vi "Port Open (SubVI).vi"(0 "VISA Refnum in":refnum<visa-resource-name>) -> (1 "VISA Refnum out":refnum<visa-resource-name>, 2 "error out":errorcluster)   [LabVIEW 2017]
doc: "by Tanguy BOULARD"
uses:
  <vilib>/Instr/_visa.llb/VISA Configure Serial Port (Instr).vi
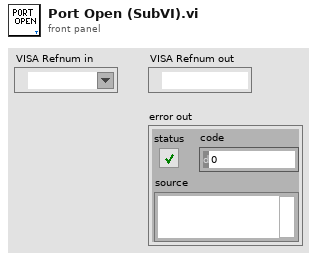
[diagram p1: front panel]
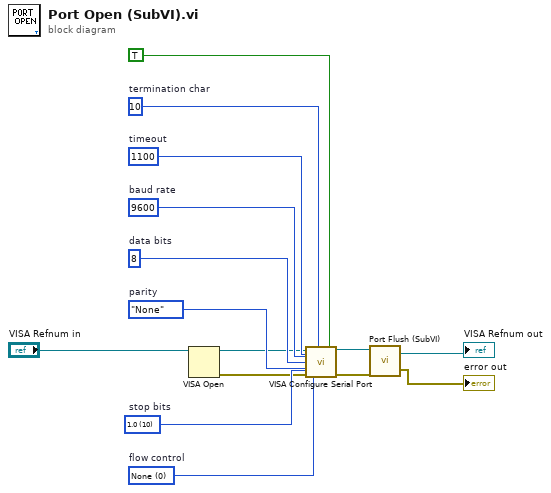
[diagram p0: block diagram]
diagram:
  w14 = u16 0 items=["None", "XON/XOFF", "RTS/CTS", "XON/XOFF & RTS/CTS", "DTR/DSR", "XON/XOFF & DTR/DSR"]  # flow control
  w13 = u16 10 items=["1.0"=10, "1.5"=15, "2.0"=20]  # stop bits
  w12 = u16 8  # data bits
  w11 = enum16{"None", "Odd", "Even", "Mark", "Space"}."None"  # parity
  w10 = u32 9600  # baud rate
  w8 = u32 1100  # timeout
  w9 = u8 10  # termination char
  n1 = VISA Open(VISA resource name="VISA Refnum in") -> (VISA resource name=w1:refnum<visa-resource-name>, error out=w2:errorcluster)  [unwired: 4 in]
  n2 = call-poly "VISA Configure Serial Port"("VISA resource name"=w1, "timeout (10sec)"=w8, "termination char\n(0xA = '\\n' = LF)"=w9, "Enable Termination\nChar (T)"=TRUE ("Enable Termination\nChar (T)"), "baud rate (9600)"=w10, "data bits (8)"=w12, "parity (0:none)"=w11, "error in (no error)"=w2, "stop bits (10: 1 bit)"=w13, "flow control (0:none)"=w14) -> ("VISA resource name out"=w6:refnum<visa-resource-name>, "error out"=w5:errorcluster)  [unwired: 4 in]
  n3 = call "Port Flush (SubVI).vi"("error in"=w5, "VISA Refnum in"=w6) -> ("error out"=→"error out":errorcluster, "VISA Refnum out"=→"VISA Refnum out":refnum<visa-resource-name>)
